vi "SQL_test_template_deletebyname.vi"(11 "模板名称":string) -> (3 "error out":errorcluster)   [LabVIEW 2014]
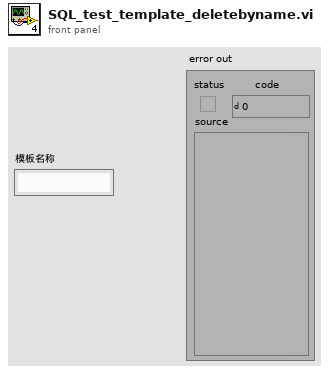
[diagram p1: front panel]
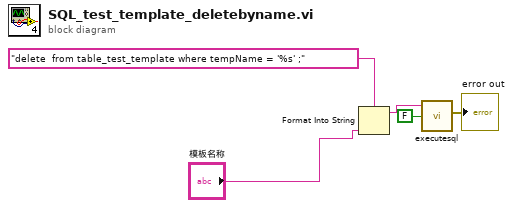
[diagram p0: block diagram]
diagram:
  n1 = Format Into String(format string="delete  from table_test_template where tempName = '%s' ;" ("Command Text"), "模板名称") -> (resulting string=w3:string)  [unwired: 2 in, 1 out]
  n2 = call "executesql.vi"("Return Data (T)"=FALSE, "Command Text"=w3) -> ("error out"=→"error out":errorcluster)  [unwired: 5 in, 1 out]
